vi "TDMS File Viewer.vi"(4 "error in (no error)":errorcluster, 7 "file path":path) -> (0 "error out":errorcluster, 3 "file path out":path)   [LabVIEW 2015]
doc: "<B>Copyright:</B> (c) 2015 National Instruments. All rights reserved.\n\nOpens the .tdms file specified in the <B>file path</B> input and presents the file data in the TDMS File Viewer dialog box."
uses:
  <vilib>/Utility/tdmsutil.llb/fileViewerConfigData.ctl
  <vilib>/Utility/error.llb/DialogType.ctl
  <vilib>/event_ctls.llb/sizeaction.ctl
  <vilib>/event_ctls.llb/panelstate.ctl
  <vilib>/Utility/tdmsutil.llb/TDMSFileViewerLocalizedText.vi
  Instance           1 26Saved   TDMS - File Viewer .vi
panel:
  in  "Load file":bool
  out "LastXScaleFormat":u8
  out "TotalCount":u64
  out "Temp Configuration":T1
  in  "LastTopLeftValue":u64
  out "Resize?":bool
  in  "Help":bool
  in  "Status":string
  in  "Quit":bool
  in  "Settings...":bool
  in  "Properties / Values / Graph":T2(tab)
  in  "Properties":i32(listbox)
  in  "Go To":bool
  in  "Scrollbar":u64(c297)
  in  "Raw data values":i32(listbox)
  out "Waveform Graph":waveform(dbl)[](graph)
  in  "File contents":string(tree)
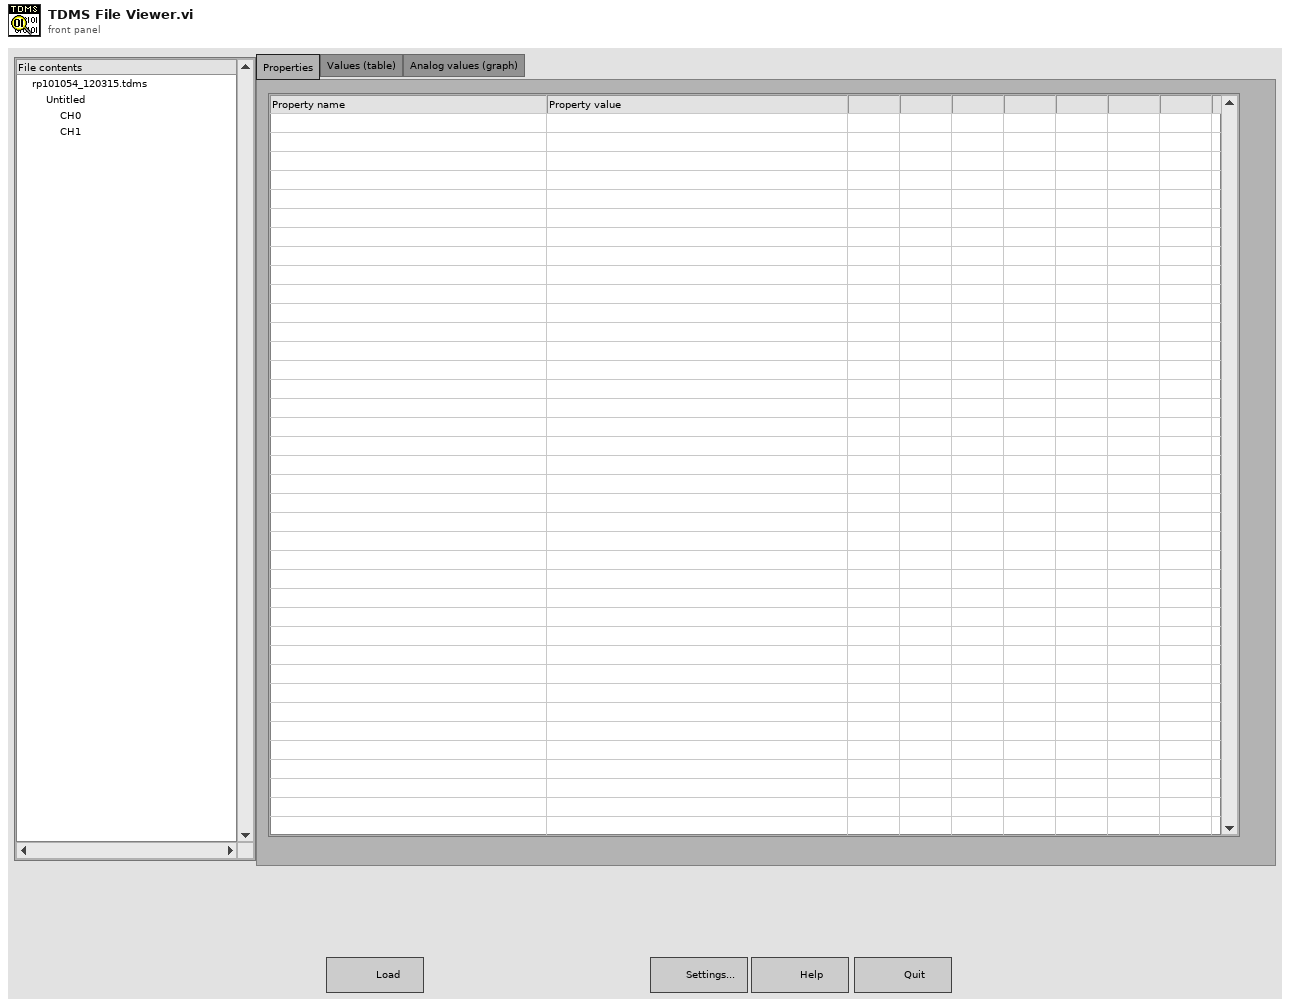
[diagram p1: front panel]
types:
  T1 = typedef "fileViewerConfigData.ctl" = cluster{"Show all (table)":bool, "Show all (graph)":bool, "limit (table)":u64, "limit (graph)":u64, "no show":bool, "start (table)":u64, "start (graph)":u64}
  T2 = enum32{"Properties", "Values (table)", "Analog values (graph)"}
  T3 = cluster{"tdms file ":refnum<k34>, "group names":string[], "channel names":string[]}[]
  T4 = cluster{"Tree":refnum<vi>, "Tab Control":refnum<vi>, "property list":refnum<vi>, "raw data list":refnum<vi>, "Waveform Graph":refnum<vi>, "Ok":refnum<vi>, "Ok 2":refnum<vi>, "Ok 3":refnum<vi>, "Ok 4":refnum<vi>, "Scrollbar":refnum<vi>, "Ok 5":refnum<vi>, "TopLeftValue":refnum<vi>, "TotalCount":refnum<vi>}
  T5 = cluster{"tdms file ":refnum<k34>, "group names":string[], "channel names":string[]}
  T6 = enum16{"open", "open or create", "create or replace", "create", "open (read-only)"}
  T7 = typedef "panelstate.ctl" = enum32{"Standard", "Minimized", "Maximized"}
  T8 = typedef "sizeaction.ctl" = enum32{"Minimized", "Maximized", "Resized"}
  T9 = cluster{"Shift":bool, "Ctrl":bool, "Alt":bool, "Cmd":bool, "Opt":bool}
  T10 = typedef "LVRectTypeDef.ctl" = cluster{"Left":i16, "Top":i16, "Right":i16, "Bottom":i16}
  T11 = typedef "LVRowAndColumnUnsignedTypeDef.ctl" = cluster{"Row":u32, "Column":u32}
  T12 = typedef "DialogType.ctl" = u16
  T13 = typedef "eventvkey.ctl" = enum16{"ASCII", "Enter", "Return", "Shift", "Ctrl", "Alt", "Cmd", "Opt", "Caps", "NumLock", "Clear", "Break", "Up", "Down", "Left", "Right", "Insert", "Delete", "Home", "End", "PageUp", "PageDown", "Escape", "Help", "Pause", "ScrollLock", "F1", "F2", "F3", "F4", "F5", "F6", "F7", "F8", "F9", "F10", "F11", "F12", "F13", "F14", "F15", "F16", "F17", "F18", "F19", "F20", "F21", "F22", "F23", "F24", "Play", "VolumeUp", "VolumeDown", "Mute", "Two Byte Char"}
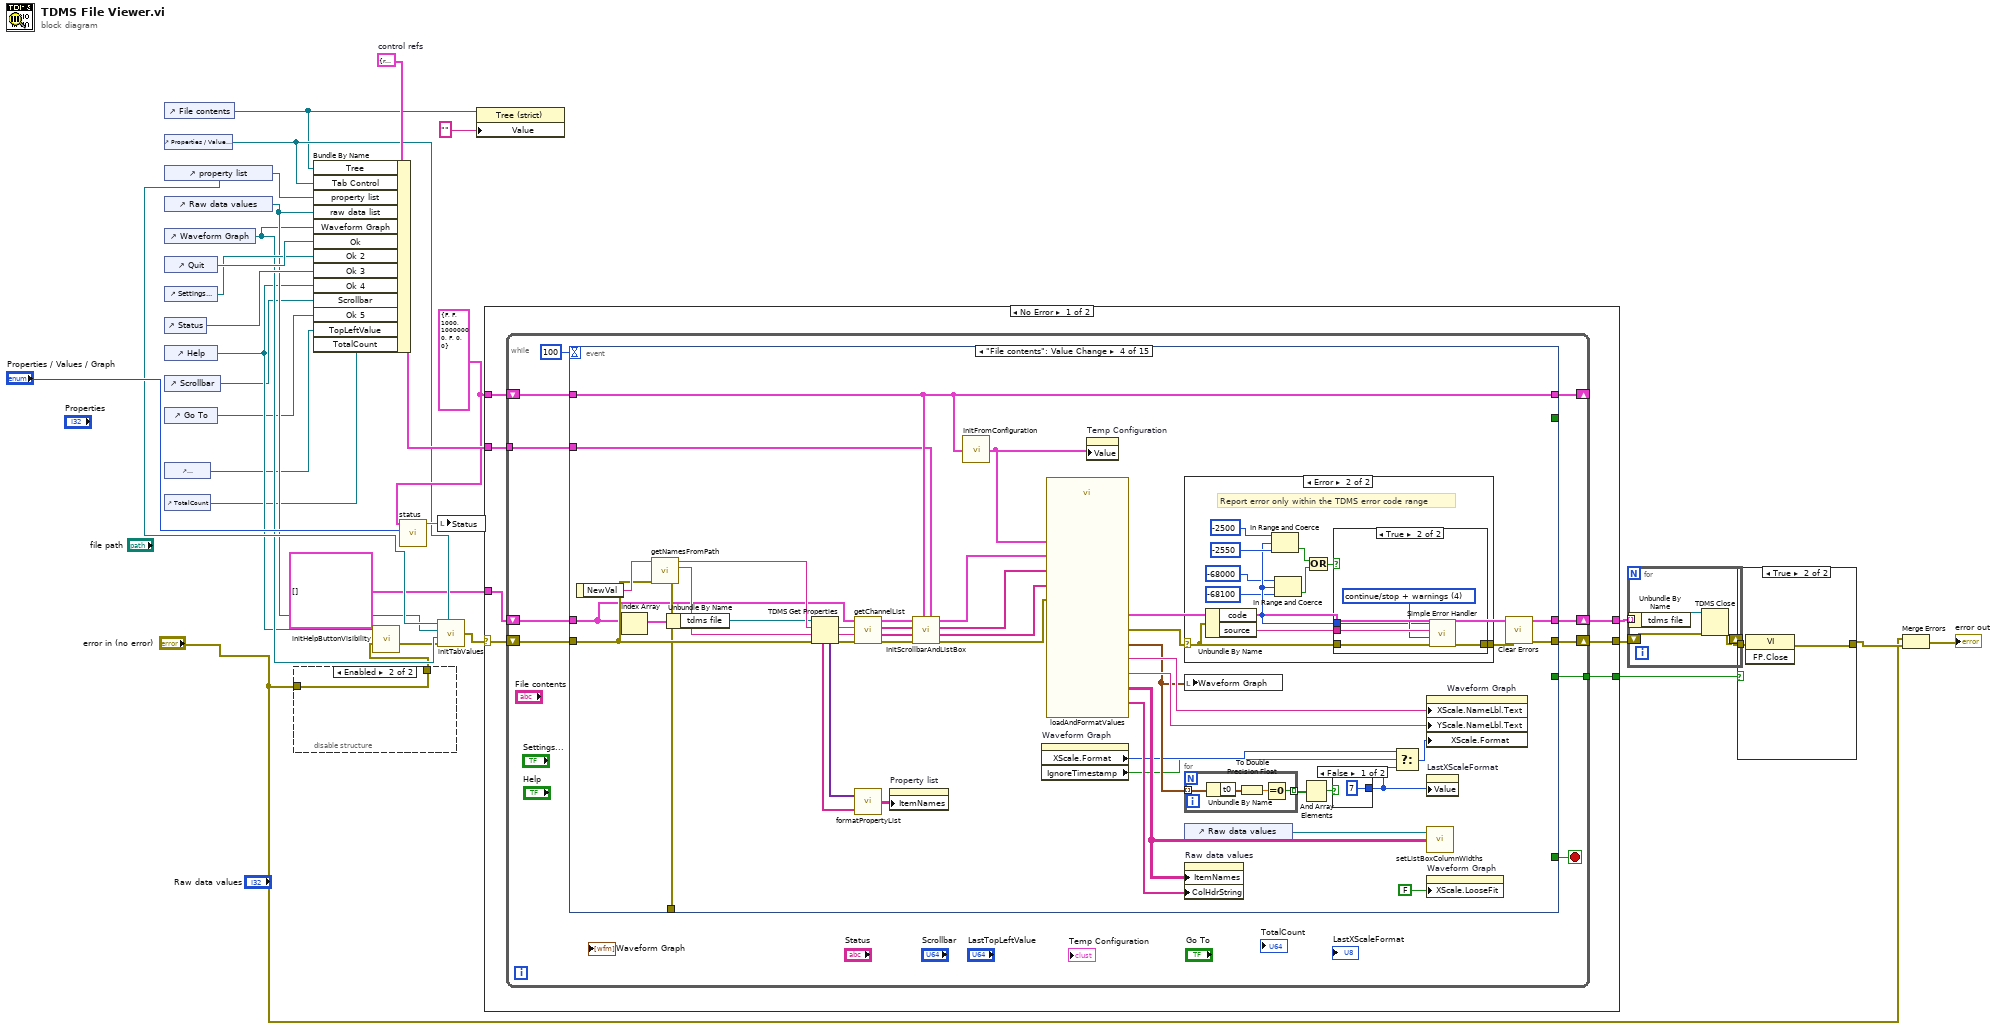
[diagram p0: block diagram]
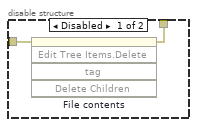
[diagram p2: hidden frame]
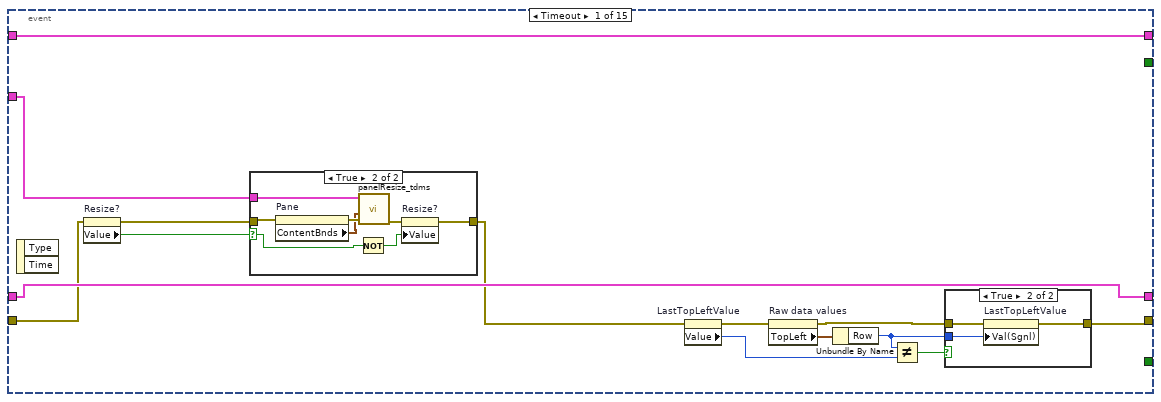
[diagram p4: hidden frame]
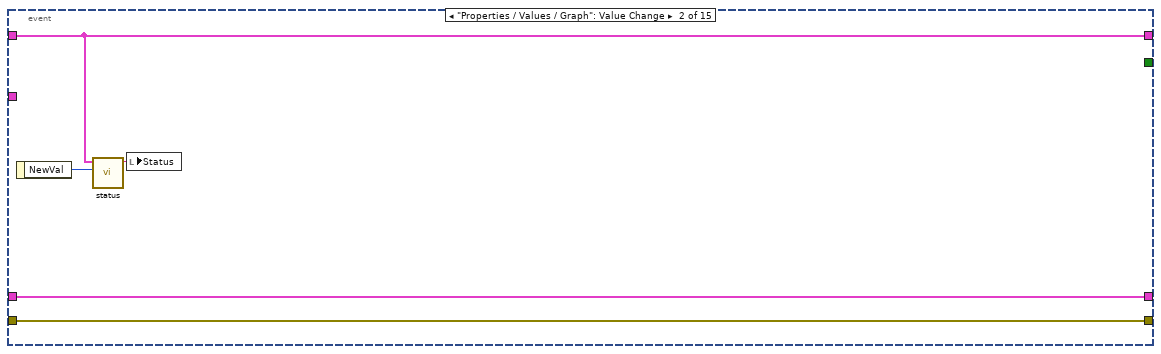
[diagram p7: hidden frame]
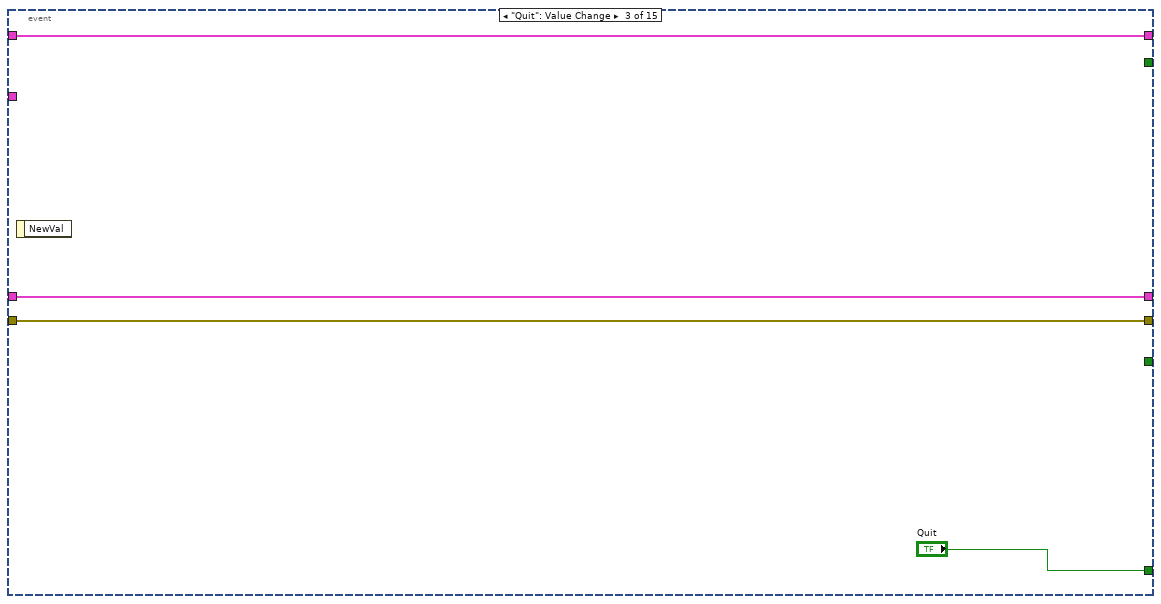
[diagram p8: hidden frame]
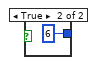
[diagram p9: hidden frame]
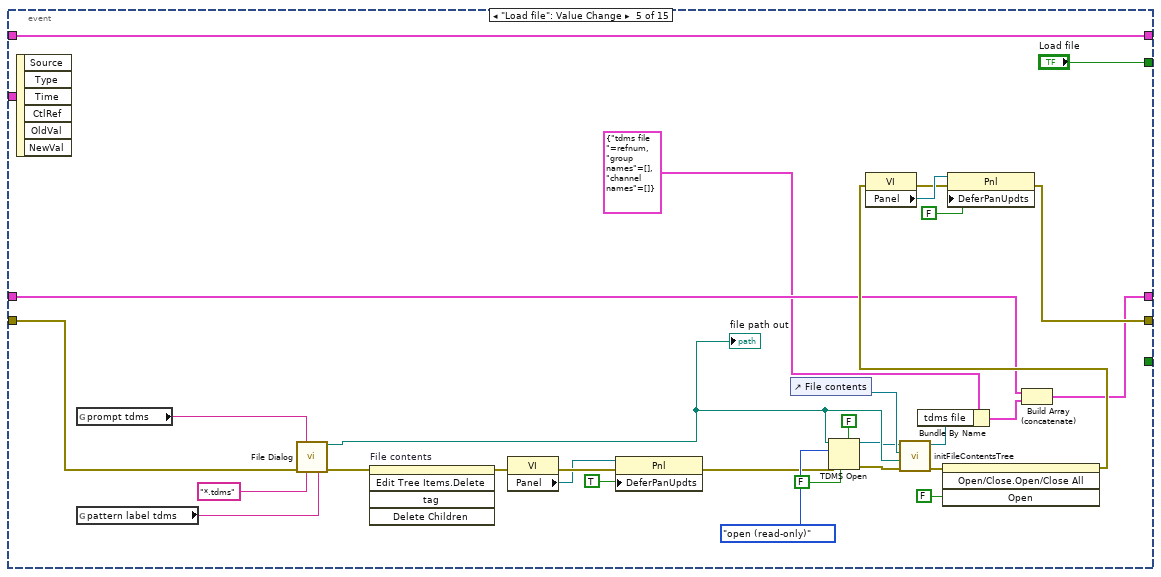
[diagram p12: hidden frame]
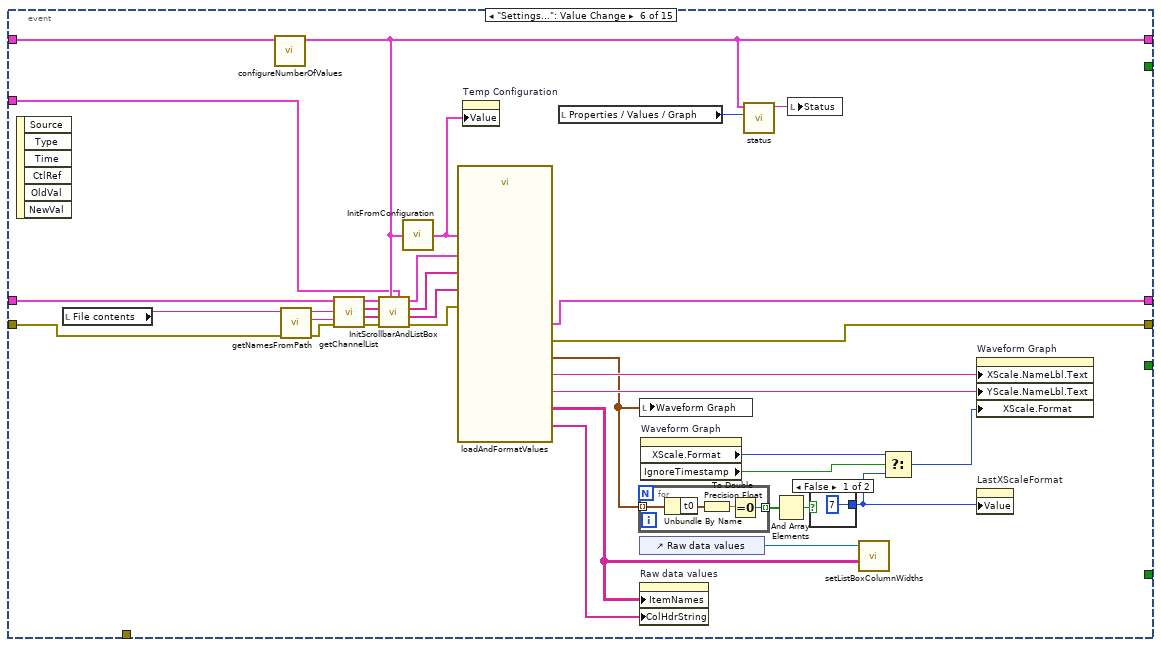
[diagram p13: hidden frame]
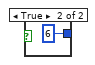
[diagram p14: hidden frame]
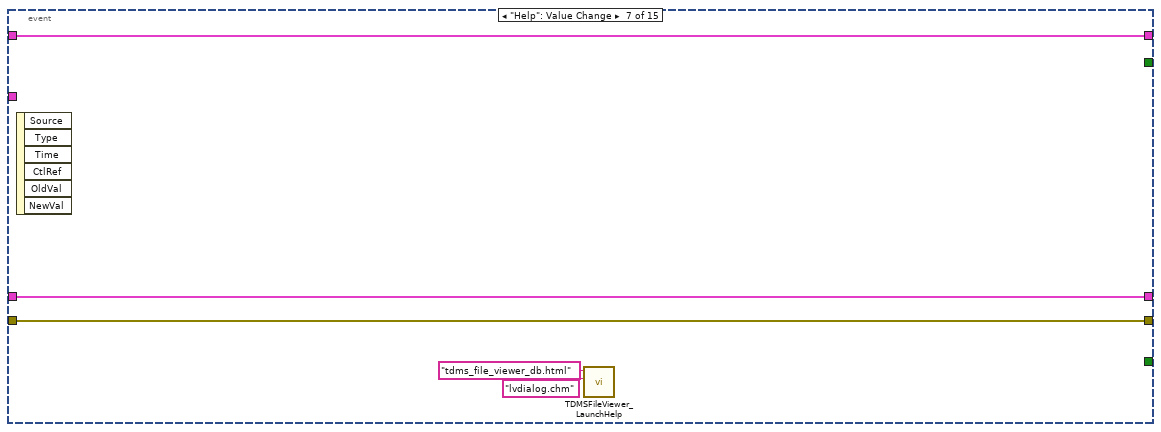
[diagram p15: hidden frame]
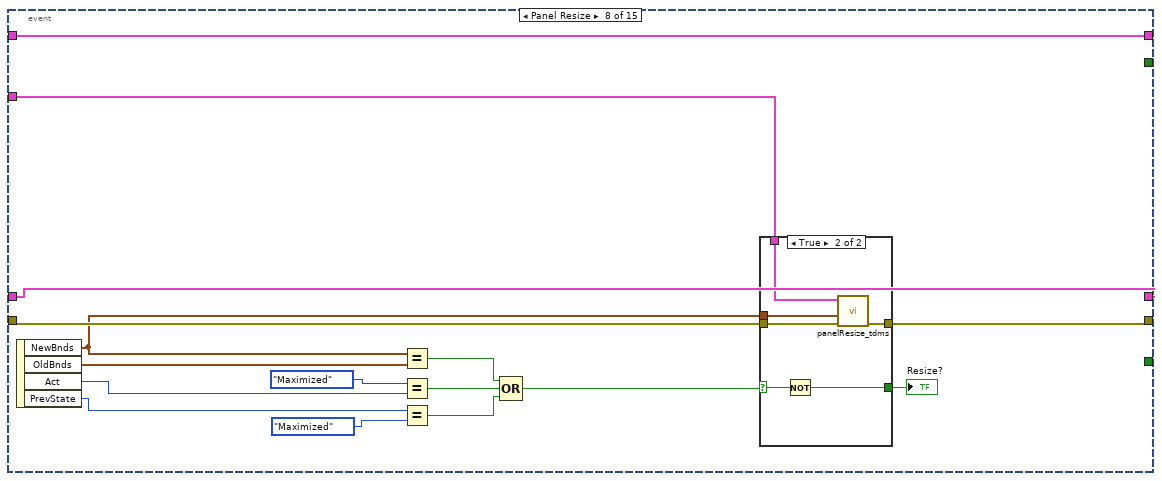
[diagram p16: hidden frame]
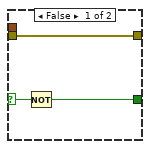
[diagram p17: hidden frame]
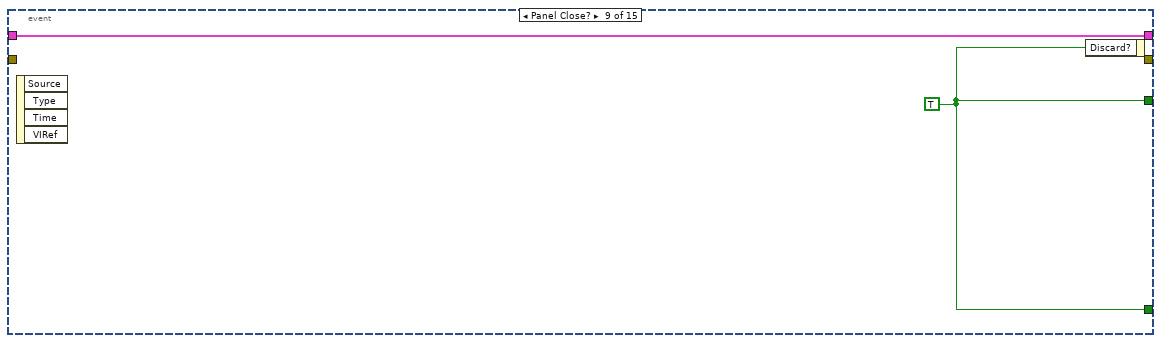
[diagram p18: hidden frame]
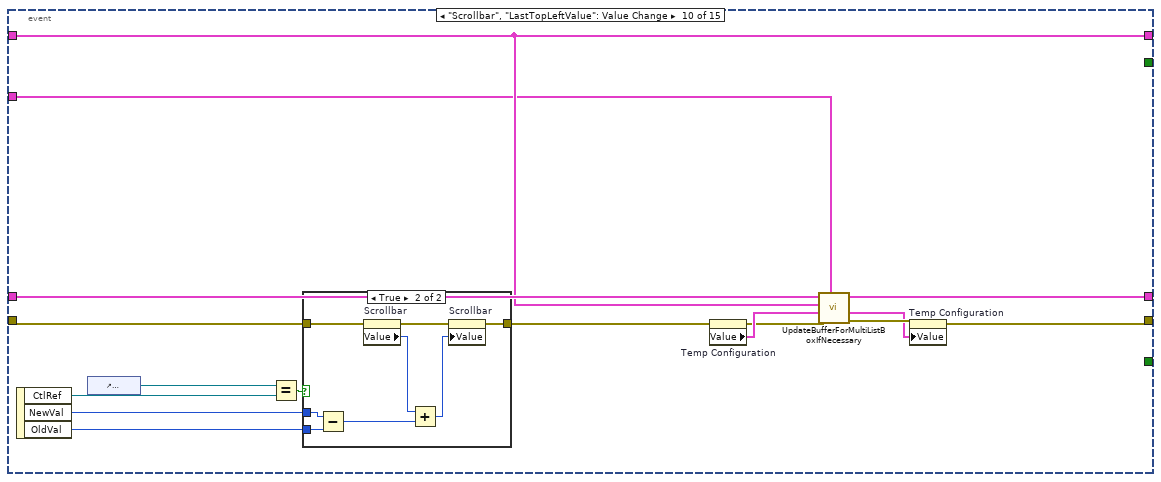
[diagram p19: hidden frame]
diagram:
  w22 = T1 {"Show all (table)"=FALSE, "Show all (graph)"=FALSE, "limit (table)"=1000, "limit (graph)"=10000000, "no show"=FALSE, "start (table)"=0, "start (graph)"=0} ("TDMS File Viewer Configuration")
  w26 = T4 {"Tree"=refnum, "Tab Control"=refnum, "property list"=refnum, "raw data list"=refnum, "Waveform Graph"=refnum, "Ok"=refnum, "Ok 2"=refnum, "Ok 3"=refnum, "Ok 4"=refnum, "Scrollbar"=refnum, "Ok 5"=refnum, "TopLeftValue"=refnum, "TotalCount"=refnum}  # control refs
  n1 = control-ref of="File contents"() -> (w13:refnum<vi>)
  n2 = control-ref of="Properties / Values / Graph"() -> (w14:refnum<vi>)
  n3 = control-ref of="property list"() -> (w17:refnum<vi>)
  n4 = control-ref of="Raw data values"() -> (w16:refnum<vi>)
  n5 = control-ref of="Waveform Graph"() -> (w15:refnum<vi>)
  n6 = control-ref of="Quit"() -> (w27:refnum<vi>)
  n7 = control-ref of="Settings..."() -> (w25:refnum<vi>)
  n8 = control-ref of="Status"() -> (w24:refnum<vi>)
  n9 = control-ref of="Help"() -> (w10:refnum<vi>)
  n10 = control-ref of="Scrollbar"() -> (w7:refnum<vi>)
  n11 = control-ref of="Go To"() -> (w6:refnum<vi>)
  n12 = control-ref of="LastTopLeftValue"() -> (w5:refnum<vi>)
  n13 = control-ref of="TotalCount"() -> (w4:refnum<vi>)
  n14 = disable-structure shown="Enabled" {
    disable-tunnel: "error in (no error)" -> [w32 w33]
    disable-tunnel: [w31 w33] -> w2
    frame Disabled {
      n15 = invoke on="File contents" class="Tree (strict)" method="Edit Tree Items.Delete"(error in=w32) -> (error out=w31:errorcluster)  [unwired: 4 in, 4 out]
    }
    frame Enabled {
    }
  }
  n16 = Bundle By Name(cluster=w26, "Tree"=w13, "Tab Control"=w14, "property list"=w17, "raw data list"=w16, "Waveform Graph"=w15, "Ok"=w27, "Ok 2"=w25, "Ok 3"=w24, "Ok 4"=w10, "Scrollbar"=w7, "Ok 5"=w6, "TopLeftValue"=w5, "TotalCount"=w4) -> (w28:T4)
  n17 = call <vilib>:"initHelpButtonVisibility.vi"("error in"=w2, "Help"=w10) -> ("error out"=w11:errorcluster)  [unwired: 9 in]
  n18 = call <vilib>:"status.vi"("tab sheet"="Properties / Values / Graph", "TDMS File Viewer Configuration"=w22) -> ("status"=w23:string)  [unwired: 5 out]
  n19 = local write "Status"(w23) -> ()
  n20 = call <vilib>:"initTabValues.vi"("properties"=w17, "Values"=w16, "waveform"=w15, "error in"=w11, "Properties / Values / Graph"=w14) -> ("error out"=w18:errorcluster)
  n21 = property class="Tree (strict)"(reference=w13, "Value"="") -> ()  [unwired: 1 in, 2 out]
  n22 = case shown="No Error" w18 {
    selector: w18 -> [w36 w389]
    tunnel: [w40 _] -> w30
    tunnel: [w39 w388] -> w29
    tunnel: w28 -> [w38 _]
    tunnel: w22 -> [w37 _]
    tunnel: [w35 FALSE] -> w20
    tunnel: T3 [] -> [w34 _]
    frame No Error {
      n23 = while {
        shift-right: [w48] -> w39
        shift-left: w36 -> [w49]
        shift-right: [w47] -> w40
        shift-left: w34 -> [w50]
        tunnel: w38 -> [w45]
        shift-right: [w43] -> _
        shift-left: w37 -> [w44]
        tunnel: [w42] -> w35
        stop <- w46 stop-if-true
        n24 = event shown="[3] \"File contents\": Value Change" {
          selector: _ -> [_ _ _ _ _ _ _ _ _ _ _ _ _ _ _]
          dyn-events: _ -> [_ _ _ _ _ _ _ _ _ _ _ _ _ _ _]
          timeout: 100 -> [_ _ _ _ _ _ _ _ _ _ _ _ _ _ _]
          tunnel: w50 -> [w64 w81 w85 w87 w157 w207 w227 w244 w255 w271 w290 w315 w330 w363 w380]
          tunnel: w49 -> [w59 w82 w84 w121 w164 w214 w226 w242 _ w258 w282 w304 w327 w362 w379]
          tunnel: [w52 w82 w84 w117 w159 w215 w226 w241 _ w265 w287 w307 w328 w362 w371] -> w48
          tunnel: [w64 w81 w85 w128 w156 w216 w227 w244 w255 w270 w289 w314 w329 w363 w380] -> w47
          tunnel: [_ _ "Quit" _ _ _ _ _ w254 _ _ _ _ _ _] -> w46
          tunnel: [_ _ _ w120 _ _ _ _ _ _ _ _ _ _ _] -> _
          tunnel: w45 -> [w60 _ _ w97 _ w191 _ w243 _ w257 w283 w305 w324 _ _]
          tunnel: w44 -> [w63 w78 w83 w98 w158 w217 w228 w240 _ w269 w291 w316 w331 w364 w381]
          tunnel: [w63 w78 w83 w98 w158 w193 w228 w240 _ w269 w291 w316 w331 w364 w381] -> w43
          tunnel: [_ _ _ _ _ _ _ _ w254 _ _ _ _ _ _] -> w42
          tunnel: [_ _ _ _ "Load file" _ _ _ _ _ _ _ _ _ _] -> _
          event Timeout {
            n25 = event-data() -> ()  [unwired: 3 out]
            n26 = property on="Resize?" class="Bool (strict)"(error in=w59) -> (error out=w61:errorcluster, "Value"=w62:bool)  [unwired: 1 in, 1 out]
            n27 = case shown="True" w62 {
              selector: w62 -> [_ w76]
              tunnel: w60 -> [_ w77]
              tunnel: w61 -> [w69 w72]
              tunnel: [w69 w74] -> w57
              frame False {
              }
              frame True {
                n28 = property on="Pane" class="Pane"(error in=w72) -> (error out=w71:errorcluster, "ContentBnds"=w70:T10)  [unwired: 1 in, 1 out]
                n29 = Not(x=w76) -> (.not. x?=w73:bool)
                n30 = call <vilib>:"panelResize_tdms.vi"("error in (no error)"=w71, "NewBnds"=w70, "control refs"=w77) -> ("error out"=w75:errorcluster)  [unwired: 4 in]
                n31 = property on="Resize?" class="Bool (strict)"(error in=w75, "Value"=w73) -> (error out=w74:errorcluster)  [unwired: 1 in, 1 out]
              }
            }
            n32 = property on="LastTopLeftValue" class="DigNum (strict)"(error in=w57) -> (error out=w56:errorcluster, "Value"=w55:u64)  [unwired: 1 in, 1 out]
            n33 = property on="Raw data values" class="MCListbox (strict)"(error in=w56) -> (error out=w53:errorcluster, "TopLeft"=w58:T11)  [unwired: 1 in, 1 out]
            n34 = Unbundle By Name(w58) -> ("Row"=w51:u32)
            n35 = Not Equal?(x=w51, y=w55) -> (x != y?=w54:bool)
            n36 = case shown="True" w54 {
              tunnel: w53 -> [w65 w68]
              tunnel: [w65 w67] -> w52
              tunnel: w51 -> [_ w66]
              frame False {
              }
              frame True {
                n37 = property on="LastTopLeftValue" class="DigNum (strict)"(error in=w68, "Val(Sgnl)"=w66) -> (error out=w67:errorcluster)  [unwired: 1 in, 1 out]
              }
            }
          }
          event "Properties / Values / Graph": Value Change {
            n38 = event-data() -> ("NewVal"=w80:T2)  [unwired: 1 out]
            n39 = call <vilib>:"status.vi"("tab sheet"=w80, "TDMS File Viewer Configuration"=w78) -> ("status"=w79:string)  [unwired: 5 out]
            n40 = local write "Status"(w79) -> ()
          }
          event "Quit": Value Change {
            n41 = event-data() -> ()  [unwired: 2 out]
          }
          event "File contents": Value Change {
            n42 = event-data() -> ("NewVal"=w123:string)  [unwired: 1 out]
            n43 = Index Array(array=w87) -> (element=w89:T5)  [unwired: 1 in]
            n44 = call "getNamesFromPath.vi"("error in (no error)"=w121, "tree path"=w123) -> ("error out"=w120:errorcluster, "channel"=w126:string, "group"=w127:string)  [unwired: 1 in, 2 out]
            n45 = Unbundle By Name(w89) -> ("tdms file"=w88:refnum<k34>)
            n46 = TDMS Get Properties(8:w121, 9:w126, 10:w127, 11:w88) -> (0:w116:errorcluster, 1:w115:string, 2:w111:string, 4:w124:variant[], 6:w125:string[])  [unwired: 3 out]
            n47 = call "getChannelList.vi"("error in (no error)"=w116, "channel names"=w115, "group name"=w111, "TDMS descriptor array"=w87) -> ("error out"=w106:errorcluster, "channel names out"=w104:string[], "group names out"=w102:string[], "TDMS descriptor array out"=w100:T3)
            n48 = call <vilib>:"formatPropertyList.vi"("property names"=w125, "property values"=w124) -> ("strings"=w122:string[][])
            n49 = property on="Property list" class="MCListbox (strict)"("ItemNames"=w122) -> ()  [unwired: 2 in, 2 out]
            n50 = call "InitScrollbarAndListBox.vi"("control refs"=w97, "configuration"=w98, "error in (no error)"=w106, "channel names"=w104, "group names"=w102, "TDMS descriptor array"=w100) -> ("error out"=w105:errorcluster, "channel out"=w103:string[], "group out"=w101:string[], "TDMS descriptor array out"=w99:T3)  [unwired: 2 in]
            n51 = call <vilib>:"InitFromConfiguration.vi"("configuration"=w98) -> ("output cluster"=w107:T1)  [unwired: 4 in]
            n52 = property on="Waveform Graph" class="WFGraph (strict)"() -> ("XScale.Format"=w91:u8, "IgnoreTimestamp"=w90:bool)  [unwired: 2 in, 2 out]
            n53 = call "loadAndFormatValues.vi"("error in (no error)"=w105, "configuration"=w107, "channel names"=w103, "group names"=w101, "TDMS descriptor array"=w99) -> ("error out"=w110:errorcluster, "graph y names"=w113:string, "graph x names"=w112:string, "TDMS descriptor array out"=w128:T3, "waveform values"=w96:waveform(dbl)[], "table values"=w119:string[][], "table headers"=w114:string[])
            n54 = property on="Temp Configuration" class="Clust (strict)"("Value"=w107) -> ()  [unwired: 2 in, 2 out]
            n55 = case shown="Error" w110 {
              selector: w110 -> [w135 w145]
              tunnel: [w135 w144] -> w109
              frame No Error {
              }
              frame Error {
                # "Report error only within the TDMS error code range"
                n56 = Unbundle By Name(w145) -> ("code"=w141:i32, "source"=w146:string)
                n57 = In Range and Coerce(upper limit=-2500, x=w141, lower limit=-2550 ("upper limit")) -> (In Range?=w138:bool)  [unwired: 1 out]
                n58 = In Range and Coerce(upper limit=-68000, x=w141, lower limit=-68100) -> (In Range?=w137:bool)  [unwired: 1 out]
                n59 = Or(x=w138, y=w137) -> (x .or. y?=w136:bool)
                n60 = case shown="True" w136 {
                  tunnel: w146 -> [_ w152]
                  tunnel: w145 -> [w147 w151]
                  tunnel: [w147 w150] -> w144
                  tunnel: w141 -> [_ w148]
                  frame False {
                    # "Out of the range of TDMS\nerror code, we don't report\nthem."
                  }
                  frame True {
                    w149 = T12 4 items=["no dialog", "OK message", "continue or stop message", "OK message + warnings", "continue/stop + warnings"] ("type of dialog (OK msg:1)")
                    n61 = call <vilib>:"Simple Error Handler.vi"("error code (no error:0)"=w148, "error source (\" \")"=w152, "type of dialog (OK msg:1)"=w149, "error in (no error)"=w151) -> ("error out"=w150:errorcluster)  [unwired: 1 in, 4 out]
                  }
                }
              }
            }
            n62 = local write "Waveform Graph"(w96) -> ()
            n63 = for {
              tunnel: w96 -> [w134] mode=indexing
              tunnel: [w131] -> w95 mode=indexing
              n64 = Unbundle By Name(w134) -> ("t0"=w133:timestamp)
              n65 = To Double Precision Float(number=w133) -> (double precision float=w132:dbl)
              n66 = Equal To 0?(x=w132) -> (x = 0?=w131:bool)
            }
            n67 = control-ref of="Raw data values"() -> (w118:refnum<vi>)
            n68 = property on="Raw data values" class="MCListbox (strict)"("ItemNames"=w119, "ColHdrString"=w114) -> ()  [unwired: 2 in, 2 out]
            n69 = And Array Elements(Boolean array=w95) -> (logical AND=w94:bool)
            n70 = case shown="False" w94 {
              tunnel: [u8 7 u8 6] -> w92
              frame False {
              }
              frame True {
              }
            }
            n71 = Select(t=w91, s=w90, f=w92) -> (s? t:f=w93:u8)
            n72 = property on="Waveform Graph" class="WFGraph (strict)"("XScale.NameLbl.Text"=w112, "YScale.NameLbl.Text"=w113, "XScale.Format"=w93) -> ()  [unwired: 2 in, 2 out]
            n73 = property on="LastXScaleFormat" class="DigNum (strict)"("Value"=w92) -> ()  [unwired: 2 in, 2 out]
            n74 = call <vilib>:"setListBoxColumnWidths.vi"("table data"=w119, "MCListbox Refnum"=w118) -> ()  [unwired: 1 out]
            n75 = property on="Waveform Graph" class="WFGraph (strict)"("XScale.LooseFit"=FALSE ("X Scale.Loose Fit")) -> ()  [unwired: 2 in, 2 out]
            n76 = call <vilib>:"Clear Errors.vi"("error in (no error)"=w109) -> ("error out"=w117:errorcluster)  [unwired: 1 in, 5 out]
          }
          event "Load file": Value Change {
            n77 = event-data() -> ()  [unwired: 7 out]
            n78 = global read "TDMSFileViewerLocalizedText.vi" "prompt tdms"() -> (w166:string)
            n79 = global read "TDMSFileViewerLocalizedText.vi" "pattern label tdms"() -> (w165:string)
            n80 = call "File Dialog"("prompt"=w166, "error in"=w164, "pattern (all files)"="*.tdms", "pattern label"=w165) -> ("selected path"=w179:path, "error out"=w180:errorcluster)  [unwired: 3 in, 7 out]
            "file path out" <- w179
            n81 = invoke on="File contents" class="Tree (strict)" method="Edit Tree Items.Delete"(error in=w180) -> (error out=w174:errorcluster)  [unwired: 4 in, 4 out]
            n82 = property class="VI"(error in=w174) -> (error out=w173:errorcluster, "Panel"=w172:refnum<vi>)  [unwired: 1 in, 1 out]
            n83 = property class="Pnl"(reference=w172, error in=w173, "DeferPanUpdts"=TRUE ("Defer Panel Updates")) -> (error out=w170:errorcluster)  [unwired: 1 out]
            n84 = control-ref of="File contents"() -> (w178:refnum<vi>)
            n85 = TDMS Open(5:FALSE ("create index file? (T)"), 6:FALSE ("disable buffering (T)"), 8:w170, 10:T6."open (read-only)" ("operation"), 11:w179) -> (0:w168:errorcluster, 3:w169:refnum<k34>)  [unwired: 2 in]
            n86 = call "initFileContentsTree.vi"("error in (no error)"=w168, "file path"=w179, "Tree Refnum"=w178, "tdms file"=w169) -> ("error out"=w175:errorcluster, "tdms file out"=w154:refnum<k34>)  [unwired: 2 out]
            n87 = Bundle By Name(cluster=T5 {"tdms file "=refnum, "group names"=[], "channel names"=[]} ("TDMS descriptor"), "tdms file"=w154) -> (w153:T5)
            n88 = invoke on="File contents" class="Tree (strict)" method="Open/Close.Open/Close All"(error in=w175, "Open"=FALSE ("Open?")) -> (error out=w160:errorcluster)  [unwired: 2 in, 3 out]
            n89 = property class="VI"(error in=w160) -> (error out=w162:errorcluster, "Panel"=w163:refnum<vi>)  [unwired: 1 in, 1 out]
            n90 = property class="Pnl"(reference=w163, error in=w162, "DeferPanUpdts"=FALSE ("Defer Panel Updates")) -> (error out=w159:errorcluster)  [unwired: 1 out]
            n91 = Build Array (concatenate)(w157, w153) -> (w156:T3)
          }
          event "Settings...": Value Change {
            n92 = event-data() -> ()  [unwired: 7 out]
            n93 = local read "File contents"() -> (w208:string)
            n94 = call <vilib>:"configureNumberOfValues.vi"("TDMS File Viewer Configuration"=w217) -> ("TDMS File Viewer Configuration Out"=w193:T1)  [unwired: 10 out]
            n95 = call "getNamesFromPath.vi"("error in (no error)"=w214, "tree path"=w208) -> ("error out"=w206:errorcluster, "channel"=w204:string, "group"=w205:string)  [unwired: 1 in, 2 out]
            n96 = call "getChannelList.vi"("error in (no error)"=w206, "channel names"=w204, "group name"=w205, "TDMS descriptor array"=w207) -> ("error out"=w195:errorcluster, "channel names out"=w197:string[], "group names out"=w199:string[], "TDMS descriptor array out"=w201:T3)
            n97 = call "InitScrollbarAndListBox.vi"("control refs"=w191, "configuration"=w193, "error in (no error)"=w195, "channel names"=w197, "group names"=w199, "TDMS descriptor array"=w201) -> ("error out"=w194:errorcluster, "channel out"=w196:string[], "group out"=w198:string[], "TDMS descriptor array out"=w200:T3)  [unwired: 2 in]
            n98 = call <vilib>:"InitFromConfiguration.vi"("configuration"=w193) -> ("output cluster"=w192:T1)  [unwired: 4 in]
            n99 = call "loadAndFormatValues.vi"("error in (no error)"=w194, "configuration"=w192, "channel names"=w196, "group names"=w198, "TDMS descriptor array"=w200) -> ("error out"=w215:errorcluster, "graph y names"=w210:string, "graph x names"=w209:string, "TDMS descriptor array out"=w216:T3, "waveform values"=w188:waveform(dbl)[], "table values"=w211:string[][], "table headers"=w213:string[])
            n100 = property on="Temp Configuration" class="Clust (strict)"("Value"=w192) -> ()  [unwired: 2 in, 2 out]
            n101 = local read "Properties / Values / Graph"() -> (w202:T2)
            n102 = for {
              tunnel: w188 -> [w223] mode=indexing
              tunnel: [w220] -> w190 mode=indexing
              n103 = Unbundle By Name(w223) -> ("t0"=w222:timestamp)
              n104 = To Double Precision Float(number=w222) -> (double precision float=w221:dbl)
              n105 = Equal To 0?(x=w221) -> (x = 0?=w220:bool)
            }
            n106 = local write "Waveform Graph"(w188) -> ()
            n107 = control-ref of="Raw data values"() -> (w212:refnum<vi>)
            n108 = property on="Raw data values" class="MCListbox (strict)"("ItemNames"=w211, "ColHdrString"=w213) -> ()  [unwired: 2 in, 2 out]
            n109 = property on="Waveform Graph" class="WFGraph (strict)"() -> ("XScale.Format"=w185:u8, "IgnoreTimestamp"=w184:bool)  [unwired: 2 in, 2 out]
            n110 = call <vilib>:"status.vi"("tab sheet"=w202, "TDMS File Viewer Configuration"=w193) -> ("status"=w203:string)  [unwired: 5 out]
            n111 = And Array Elements(Boolean array=w190) -> (logical AND=w189:bool)
            n112 = local write "Status"(w203) -> ()
            n113 = case shown="False" w189 {
              tunnel: [u8 7 u8 6] -> w186
              frame False {
              }
              frame True {
              }
            }
            n114 = call <vilib>:"setListBoxColumnWidths.vi"("table data"=w211, "MCListbox Refnum"=w212) -> ()  [unwired: 1 out]
            n115 = Select(t=w185, s=w184, f=w186) -> (s? t:f=w187:u8)
            n116 = property on="Waveform Graph" class="WFGraph (strict)"("XScale.NameLbl.Text"=w209, "YScale.NameLbl.Text"=w210, "XScale.Format"=w187) -> ()  [unwired: 2 in, 2 out]
            n117 = property on="LastXScaleFormat" class="DigNum (strict)"("Value"=w186) -> ()  [unwired: 2 in, 2 out]
          }
          event "Help": Value Change {
            n118 = event-data() -> ()  [unwired: 7 out]
            n119 = call <vilib>:"TDMSFileViewer_LaunchHelp.vi"("CHM or HLP filename (lvdialog.chm)"="lvdialog.chm", "HTML filename"="tdms_file_viewer_db.html") -> ()  [unwired: 1 in, 5 out]
          }
          event Panel Resize {
            n120 = event-data() -> ("NewBnds"=w232:T10, "OldBnds"=w231:T10, "Act"=w233:T8, "PrevState"=w234:T7)  [unwired: 1 out]
            n121 = Equal?(x=w232, y=w231) -> (x = y?=w237:bool)
            n122 = Equal?(x=sizeaction."Maximized" ("Act"), y=w233) -> (x = y?=w236:bool)
            n123 = Equal?(x=w234, y=panelstate."Maximized" ("PrevState")) -> (x = y?=w235:bool)
            n124 = Compound Arithmetic op=OR(w237, w236, w235) -> (w230:bool)
            n125 = case shown="True" w230 {
              selector: w230 -> [w246 w249]
              tunnel: w243 -> [_ w253]
              tunnel: w242 -> [w247 w252]
              tunnel: [w247 w251] -> w241
              tunnel: w232 -> [_ w250]
              tunnel: [w245 w248] -> w229
              frame False {
                n126 = Not(x=w246) -> (.not. x?=w245:bool)
              }
              frame True {
                n127 = Not(x=w249) -> (.not. x?=w248:bool)
                n128 = call <vilib>:"panelResize_tdms.vi"("error in (no error)"=w252, "NewBnds"=w250, "control refs"=w253) -> ("error out"=w251:errorcluster)  [unwired: 4 in]
              }
            }
            "Resize?" <- w229
          }
          event Panel Close? {
            w254 = TRUE
            n129 = event-data() -> ()  [unwired: 5 out]
            n130 = event-data("Discard?"=w254) -> ()  [unwired: 1 in, 1 out]
          }
          event "Scrollbar", "LastTopLeftValue": Value Change {
            n131 = event-data() -> ("CtlRef"=w263:refnum<vi>, "NewVal"=w260:u64, "OldVal"=w259:u64)  [unwired: 1 out]
            n132 = control-ref of="LastTopLeftValue"() -> (w262:refnum<vi>)
            n133 = Equal?(x=w262, y=w263) -> (x = y?=w261:bool)
            n134 = case shown="True" w261 {
              tunnel: w260 -> [_ w276]
              tunnel: w259 -> [_ w275]
              tunnel: w258 -> [w272 w274]
              tunnel: [w272 w273] -> w256
              frame False {
              }
              frame True {
                n135 = Subtract(x=w276, y=w275) -> (x-y=w278:u64)
                n136 = property on="Scrollbar" class="Scroll (strict)"(error in=w274) -> (error out=w280:errorcluster, "Value"=w279:u64)  [unwired: 1 in, 1 out]
                n137 = Add(x=w279, y=w278) -> (x+y=w277:u64)
                n138 = property on="Scrollbar" class="Scroll (strict)"(error in=w280, "Value"=w277) -> (error out=w273:errorcluster)  [unwired: 1 in, 1 out]
              }
            }
            n139 = property on="Temp Configuration" class="Clust (strict)"(error in=w256) -> (error out=w267:errorcluster, "Value"=w268:T1)  [unwired: 1 in, 1 out]
            n140 = call "UpdateBufferForMultiListBoxIfNecessary.vi"("control refs"=w257, "error in"=w267, "Buffer Configuration"=w268, "TDMS File Viewer Configuration"=w269, "TDMS descriptor array"=w271) -> ("error out"=w266:errorcluster, "BufferConfig out"=w264:T1, "TDMS descriptor array out"=w270:T3)  [unwired: 4 in]
            n141 = property on="Temp Configuration" class="Clust (strict)"(error in=w266, "Value"=w264) -> (error out=w265:errorcluster)  [unwired: 1 in, 1 out]
          }
          event "Raw data values": Key Down?; "Raw data values": event type 3.0.x8000000b {
            n142 = event-data() -> ("VKey"=w285:T13)  [unwired: 1 out]
            n143 = call <vilib>:"UpdateScrollbarBeforeKeyEvent.vi"("error in (no error)"=w282, "VKey"=w285, "control refs 2"=w283) -> ("error out"=w288:errorcluster, "LoadBuffer?"=w286:bool, "DiscardEvent?"=w284:bool)  [unwired: 6 in]
            n144 = case shown="True" w286 {
              tunnel: w291 -> [_ w299]
              tunnel: w290 -> [w292 w298]
              tunnel: [w292 w297] -> w289
              tunnel: w288 -> [w293 w294]
              tunnel: [w293 w296] -> w281
              tunnel: w283 -> [_ w295]
              frame False {
              }
              frame True {
                n145 = property on="Temp Configuration" class="Clust (strict)"(error in=w294) -> (error out=w302:errorcluster, "Value"=w303:T1)  [unwired: 1 in, 1 out]
                n146 = call "UpdateBufferForMultiListBoxIfNecessary.vi"("control refs"=w295, "error in"=w302, "Buffer Configuration"=w303, "TDMS File Viewer Configuration"=w299, "TDMS descriptor array"=w298) -> ("error out"=w301:errorcluster, "BufferConfig out"=w300:T1, "TDMS descriptor array out"=w297:T3)  [unwired: 4 in]
                n147 = property on="Temp Configuration" class="Clust (strict)"(error in=w301, "Value"=w300) -> (error out=w296:errorcluster)  [unwired: 1 in, 1 out]
              }
            }
            n148 = call <vilib>:"UpdateListBoxAfterKeyEvent.vi"("DiscardEvent?"=w284, "error in (no error)"=w281, "VKey"=w285, "control refs"=w283) -> ("error out"=w287:errorcluster)  [unwired: 7 in]
            n149 = event-data("Discard?"=w284) -> ()  [unwired: 1 in, 1 out]
          }
          event "Go To": Value Change {
            n150 = event-data() -> ()  [unwired: 2 out]
            n151 = call <vilib>:"GoTo.vi"("error in"=w304, "control refs"=w305) -> ("error out"=w313:errorcluster, "VisibleValue"=w310:u64)  [unwired: 8 in]
            n152 = property on="Temp Configuration" class="Clust (strict)"(error in=w313) -> (error out=w319:errorcluster, "Value"=w320:T1)  [unwired: 1 in, 1 out]
            n153 = call "UpdateBufferForMultiListBoxIfNecessary.vi"("control refs"=w305, "error in"=w319, "Buffer Configuration"=w320, "TDMS File Viewer Configuration"=w316, "TDMS descriptor array"=w315) -> ("error out"=w318:errorcluster, "BufferConfig out"=w317:T1, "TDMS descriptor array out"=w314:T3)  [unwired: 4 in]
            n154 = property on="Temp Configuration" class="Clust (strict)"(error in=w318, "Value"=w317) -> (error out=w306:errorcluster)  [unwired: 1 in, 1 out]
            n155 = property on="Raw data values" class="MCListbox (strict)"(error in=w306) -> (error out=w308:errorcluster, "TopLeft"=w312:T11)  [unwired: 1 in, 1 out]
            n156 = Unbundle By Name(w312) -> ("Row"=w311:u32)
            n157 = Add(x=w311, y=w310) -> (x+y=w309:u64)
            n158 = property on="Raw data values" class="MCListbox (strict)"(error in=w308, "Value"=w309) -> (error out=w307:errorcluster)  [unwired: 1 in, 1 out]
          }
          event Key Down {
            n159 = event-data() -> ("PlatMods"=w323:T9, "Char"=w322:i16)  [unwired: 1 out]
            n160 = property on="Raw data values" class="MCListbox (strict)"(error in=w327) -> (error out=w321:errorcluster, "Key Focus"=w326:bool)  [unwired: 1 in, 1 out]
            n161 = case shown="True" w326 {
              selector: w326 -> [w332 _]
              tunnel: [w332 w333] -> w325
              tunnel: w323 -> [_ w338]
              tunnel: w322 -> [_ w337]
              frame False {
              }
              frame True {
                n162 = disable-structure shown="Default" {
                  disable-tunnel: [T9 {"Shift"=FALSE, "Ctrl"=TRUE, "Alt"=FALSE, "Cmd"=FALSE, "Opt"=TRUE} ("PlatMods") T9 {"Shift"=FALSE, "Ctrl"=FALSE, "Alt"=FALSE, "Cmd"=TRUE, "Opt"=FALSE} ("PlatMods")] -> w339
                  frame condition #0 (active) {
                  }
                  frame condition #1 {
                  }
                }
                n163 = Equal?(x=w339, y=w338) -> (x = y?=w335:bool)
                n164 = Equal?(x=w337, y=i16 103 ("Char")) -> (x = y?=w334:bool)
                n165 = And(x=w335, y=w334) -> (x .and. y?=w333:bool)
              }
            }
            n166 = case shown="True" w325 {
              tunnel: w331 -> [_ w357]
              tunnel: w330 -> [w342 w356]
              tunnel: [w342 w355] -> w329
              tunnel: [w343 w348] -> w328
              tunnel: w321 -> [w343 w344]
              tunnel: w324 -> [_ w346]
              tunnel: w324 -> [_ w345]
              frame False {
              }
              frame True {
                n167 = call <vilib>:"GoTo.vi"("error in"=w344, "control refs"=w345) -> ("error out"=w354:errorcluster, "VisibleValue"=w351:u64)  [unwired: 8 in]
                n168 = property on="Temp Configuration" class="Clust (strict)"(error in=w354) -> (error out=w360:errorcluster, "Value"=w361:T1)  [unwired: 1 in, 1 out]
                n169 = call "UpdateBufferForMultiListBoxIfNecessary.vi"("control refs"=w346, "error in"=w360, "Buffer Configuration"=w361, "TDMS File Viewer Configuration"=w357, "TDMS descriptor array"=w356) -> ("error out"=w359:errorcluster, "BufferConfig out"=w358:T1, "TDMS descriptor array out"=w355:T3)  [unwired: 4 in]
                n170 = property on="Temp Configuration" class="Clust (strict)"(error in=w359, "Value"=w358) -> (error out=w347:errorcluster)  [unwired: 1 in, 1 out]
                n171 = property on="Raw data values" class="MCListbox (strict)"(error in=w347) -> (error out=w349:errorcluster, "TopLeft"=w353:T11)  [unwired: 1 in, 1 out]
                n172 = Unbundle By Name(w353) -> ("Row"=w352:u32)
                n173 = Add(x=w352, y=w351) -> (x+y=w350:u64)
                n174 = property on="Raw data values" class="MCListbox (strict)"(error in=w349, "Value"=w350) -> (error out=w348:errorcluster)  [unwired: 1 in, 1 out]
              }
            }
          }
          event Key Down? {
            n175 = event-data() -> ("VKey"=w366:T13)  [unwired: 1 out]
            n176 = case shown="\"F1\"" w366 {
              tunnel: [FALSE ("Discard?") TRUE ("Discard?")] -> w365
              frame Default {
              }
              frame "F1" {
                n177 = call <vilib>:"TDMSFileViewer_LaunchHelp.vi"("CHM or HLP filename (lvdialog.chm)"="lvdialog.chm", "HTML filename"="tdms_file_viewer_db.html") -> ()  [unwired: 1 in, 5 out]
              }
            }
            n178 = event-data("Discard?"=w365) -> ()  [unwired: 1 in, 1 out]
          }
          event "Waveform Graph": Shortcut Menu Selection (App) {
            n179 = event-data() -> ("ItemTag"=w377:string)  [unwired: 1 out]
            n180 = property on="Waveform Graph" class="WFGraph (strict)"(error in=w379) -> (error out=w372:errorcluster, "IgnoreTimestamp"=w376:bool)  [unwired: 1 in, 1 out]
            n181 = Not(x=w376) -> (.not. x?=w373:bool)
            n182 = Equal?(x=w377, y="APP_SC_IGNORE_TIME_STAMP") -> (x = y?=w374:bool)
            n183 = And(x=w373, y=w374) -> (x .and. y?=w375:bool)
            n184 = case shown="True" w375 {
              tunnel: w372 -> [w382 w386]
              tunnel: [w382 w383] -> w371
              frame False {
              }
              frame True {
                n185 = property on="LastXScaleFormat" class="DigNum (strict)"(error in=w386) -> (error out=w385:errorcluster, "Value"=w384:u8)  [unwired: 1 in, 1 out]
                n186 = property on="Waveform Graph" class="WFGraph (strict)"(error in=w385, "XScale.Format"=w384) -> (error out=w383:errorcluster)  [unwired: 1 in, 1 out]
              }
            }
          }
        }
      }
    }
    frame Error {
      n187 = call <vilib>:"Simple Error Handler.vi"("error in (no error)"=w389) -> ("error out"=w388:errorcluster)  [unwired: 1 in, 7 out]
    }
  }
  n188 = for {
    tunnel: w30 -> [w393] mode=indexing
    shift-right: [w391] -> w19
    shift-left: w29 -> [w392]
    n189 = Unbundle By Name(w393) -> ("tdms file"=w390:refnum<k34>)
    n190 = TDMS Close(8:w392, 11:w390) -> (0:w391:errorcluster)  [unwired: 1 out]
  }
  n191 = case shown="True" w20 {
    tunnel: w19 -> [w394 w396]
    tunnel: [w394 w395] -> w9
    frame False {
    }
    frame True {
      n192 = invoke class="VI" method="FP.Close"(error in=w396) -> (error out=w395:errorcluster)  [unwired: 2 in, 2 out]
    }
  }
  n193 = Merge Errors("error in (no error)", w9) -> (→"error out":errorcluster)
